vi "Read Lab Laser Transmission Spectrum.vi"() -> ()   [LabVIEW 2013]
uses:
  <vilib>/Utility/file.llb/Read From Spreadsheet File (DBL).vi
panel:
  out "subarray":dbl[](array[numeric])
  in  "Frame Number":i32
  out "Original Data Graph":cluster{i32[], dbl[]}(graph)
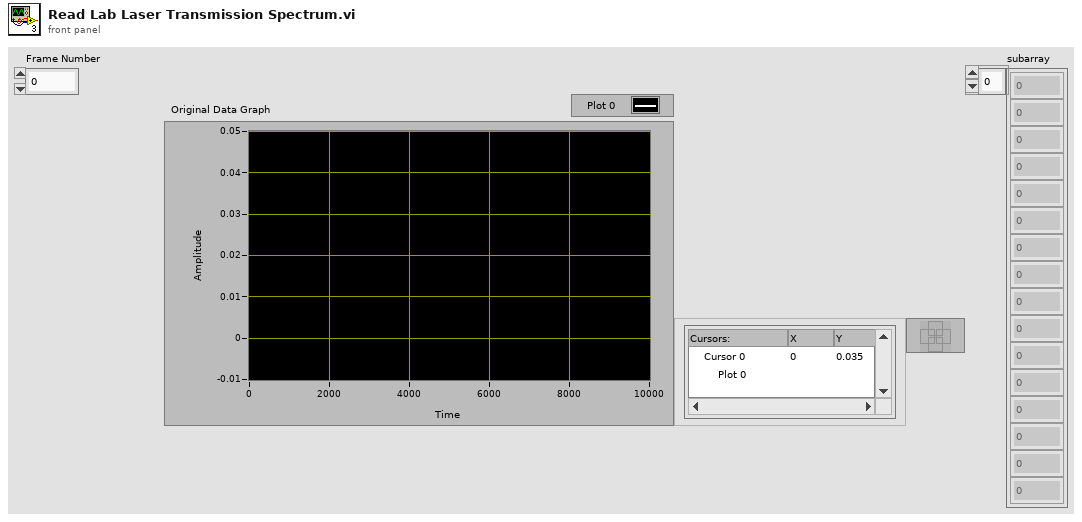
[diagram p1: front panel]
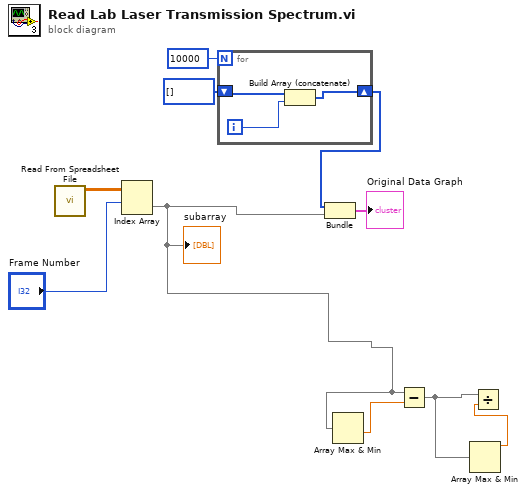
[diagram p0: block diagram]
diagram:
  n1 = call-poly <vilib>:"Read From Spreadsheet File.vi"() -> ("all rows"=w9:dbl[][])  [unwired: 7 in, 4 out]
  n2 = Index Array(array=w9, index (row)="Frame Number") -> (element=w1:dbl[])  [unwired: 1 in]
  "subarray" <- w1
  n3 = for {
    N: 10000 -> [_]
    shift-right: [w12] -> w2
    shift-left: i32[] [] -> [w11]
    i -> [w13]
    n4 = Build Array (concatenate)(w11, w13) -> (w12:i32[])
  }
  n5 = Bundle(w2, "all rows"=w1) -> (→"Original Data Graph":cluster{i32[], "all rows":dbl[]})  [unwired: 1 in]
  n6 = Array Max & Min(array=w1) -> (min value=w7:dbl)  [unwired: 3 out]
  n7 = Subtract(x=w1, y=w7) -> (x-y=w6:dbl[])
  n8 = Array Max & Min(array=w6) -> (max value=w5:dbl)  [unwired: 3 out]
  n9 = Divide(x=w6, y=w5) -> ()  [unwired: 1 out]
